vi "GT Laser Out Frq.vi"(8 "error in (no error)":errorcluster caption="错误输入（无错误）", 9 "channel":i16, 10 "outFrq":dbl, 11 "cardNum":i16) -> (0 "error out":errorcluster caption="错误输出", 3 "function return":i16)   [LabVIEW 2020, in "gts.lvlib"]
doc: "GT_API GT_LaserOutFrq(short cardNum,double outFrq,short channel=0);"
uses:
  gts.lvlib
  dll/32bit/multi_card/gts.dll
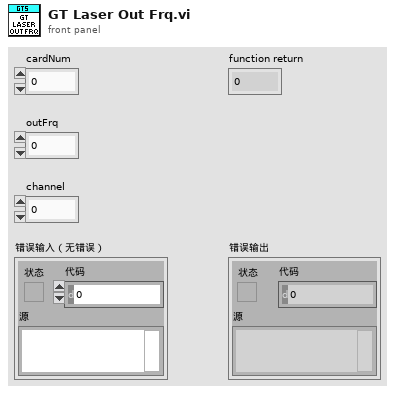
[diagram p1: front panel]
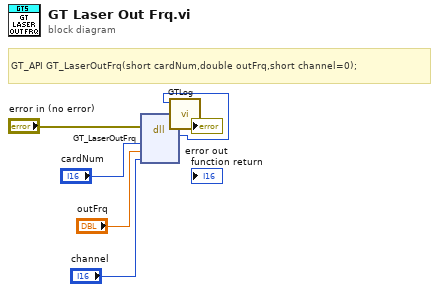
[diagram p0: block diagram]
diagram:
  # "GT_API GT_LaserOutFrq(short cardNum,double outFrq,short channel=0);"
  n1 = dll-call lib="C:/1228/dll/32bit/multi_card/gts.dll" fn="GT_LaserOutFrq"(error in="error in (no error)", "cardNum"="cardNum", "outFrq"="outFrq", "channel"="channel") -> (error out=w3:errorcluster, w1:i16)  [unwired: 5 in, 1 out]
  n2 = call "GTLog.vi"("error in (no error)"=w3, "Numeric"=w1) -> ("error out"=→"error out":errorcluster)  [unwired: 9 in]
